vi "Binomial Noise.vi"(7 "initialize?":bool=TRUE, 8 "seed":i32=-1, 9 "trial probability":dbl=0.5 format="%.2f", 10 "trials":i32=1, 11 "samples":i32=128) -> (0 "error":i32, 3 "binomial noise":u32[](array[numeric]))   [LabVIEW 2010, in "NI_AALBase.lvlib"]
doc: "Generates a binomially-distributed, pseudorandom pattern whose values are the number of occurrences of an event, given the probability of that event occurring and the number of trials."
uses:
  NI_AALBase.lvlib
  lvanlys.dll
panel:
  # "Binomial Noise"
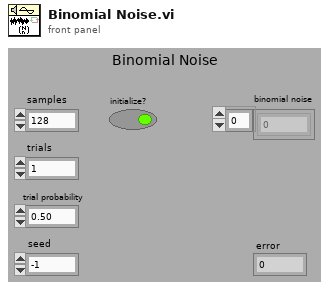
[diagram p1: front panel]
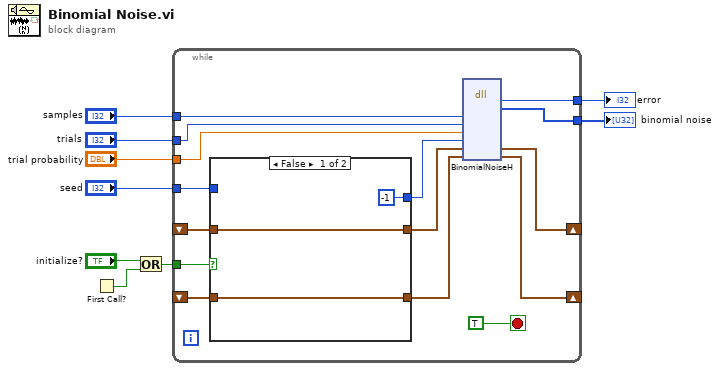
[diagram p0: block diagram]
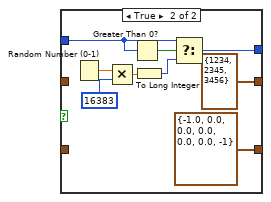
[diagram p2: hidden frame]
diagram:
  n1 = First Call?() -> (First Call?: T/F=w3:bool)
  n2 = Or(x="initialize?", y=w3) -> (x .or. y?=w2:bool)
  n3 = while {
    tunnel: [w21] -> w9
    tunnel: "seed" -> [w18]
    tunnel: "trials" -> [w24]
    tunnel: "samples" -> [w23]
    shift-right: [w10] -> _
    shift-left: _ -> [w19]
    shift-right: [w15] -> _
    shift-left: _ -> [w17]
    tunnel: w2 -> [w20]
    tunnel: "trial probability" -> [w12]
    tunnel: [w11] -> w1
    stop <- TRUE stop-if-true
    n4 = case shown="False" w20 {
      tunnel: w19 -> [w27 _]
      tunnel: [w27 cluster{"xSeed":i32, "ySeed":i32, "zSeed":i32} {"xSeed"=1234, "ySeed"=2345, "zSeed"=3456} ("RNGState")] -> w14
      tunnel: [-1 ("seed") w34] -> w13
      tunnel: w18 -> [_ w35]
      tunnel: [w26 cluster{dbl, dbl, dbl, dbl, dbl, dbl, i32} {-1.0, 0.0, 0.0, 0.0, 0.0, 0.0, -1}] -> w16
      tunnel: w17 -> [w26 _]
      frame False {
      }
      frame True {
        n5 = Random Number (0-1)() -> (number: 0 to 1=w32:dbl)
        n6 = Multiply(x=w32, y=16383 ("x")) -> (x*y=w33:dbl)
        n7 = Greater Than 0?(x=w35) -> (x > 0?=w36:bool)
        n8 = To Long Integer(number=w33) -> (32bit integer=w31:i32)
        n9 = Select(t=w35, s=w36, f=w31) -> (s? t:f=w34:i32)
      }
    }
    n10 = dll-call lib="C:/Program Files/National Instruments/LabVIEW 2010/resource/lvanlys.*" fn="BinomialNoiseH"("size"=w23, "numTrials"=w24, "trialProb"=w12, "theSeed"=w13, "rngState"=w14, "binomialState"=w16) -> ("return type"=w21:i32, "xH"=w11:u32[], "rngState"=w10:cluster{"xSeed":i32, "ySeed":i32, "zSeed":i32}, "binomialState"=w15:cluster{dbl, dbl, dbl, dbl, dbl, dbl, i32})  [unwired: 7 in, 3 out]
  }
  "error" <- w9
  "binomial noise" <- w1
